vi "Set Font.vi"(8 "error in (no error)":errorcluster, 10 "Name":string="Calibri", 11 "Style in":refnum<class "Style.lvclass">) -> (0 "error out":errorcluster, 3 "Style out":refnum<class "Style.lvclass">)   [LabVIEW 2017, in "Styles.lvlib" / "Style.lvclass"]
uses:
  Style.lvclass
  Style.lvclass/Style.ctl
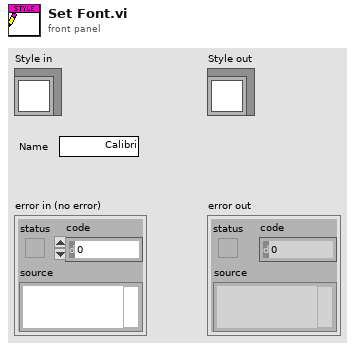
[diagram p1: front panel]
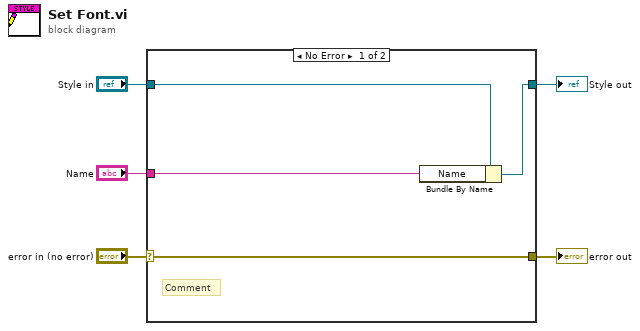
[diagram p0: block diagram]
diagram:
  n1 = case shown="No Error" "error in (no error)" {
    selector: "error in (no error)" -> [w9 w10]
    tunnel: [w9 w10] -> w4
    tunnel: [w7 w11] -> w2
    tunnel: "Style in" -> [w8 w11]
    tunnel: "Name" -> [w6 _]
    frame No Error {
      # "Comment"
      n2 = Bundle By Name(cluster=w8, "Name"=w6) -> (w7:refnum<class "Style.lvclass">)
    }
    frame Error {
    }
  }
  "error out" <- w4
  "Style out" <- w2
